vi "FYP_VI_MIDI_Test_InstrumentNote.vi"() -> ()   [LabVIEW 2013]
panel:
  in  "Pitch Note":u32=60 max=127
  in  "Velocity / Volume":u32(knob)=127 max=127 scale=0.0..127.0
  in  "stop":bool
  in  "Instrument":u32 max=127
  in  "MIDI Channel":u32 max=15
  in  "deviceID":u32
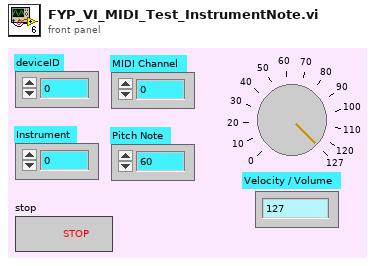
[diagram p1: front panel]
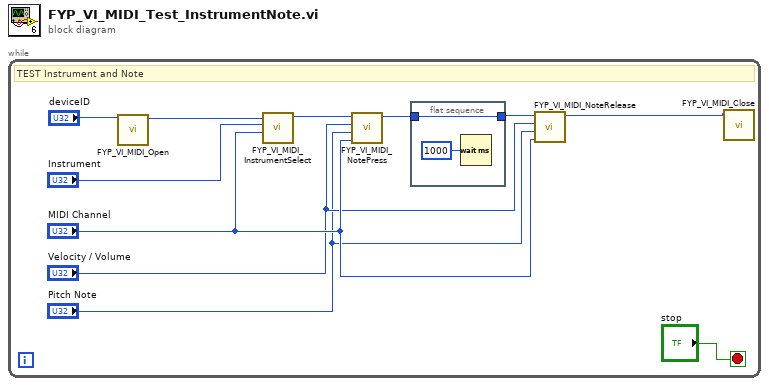
[diagram p0: block diagram]
diagram:
  n1 = while {
    stop <- "stop" stop-if-true
    # "TEST Instrument and Note"
    n2 = call "FYP_VI_MIDI_Open.vi"("deviceID"="deviceID") -> ("midiOut"=w6:i32)  [unwired: 5 in, 1 out]
    n3 = call "FYP_VI_MIDI_InstrumentSelect.vi"("MIDI Channel"="MIDI Channel", "Instrument"="Instrument", "midiOut handle"=w6) -> ("midiOut handle"=w4:i32)  [unwired: 3 in, 1 out]
    n4 = call "FYP_VI_MIDI_NotePress.vi"("MIDI Channel"="MIDI Channel", "Pitch Note"="Pitch Note", "Velocity / Volume"="Velocity / Volume", "midiOut Handle"=w4) -> ("midiOut handle"=w3:i32)  [unwired: 2 in, 1 out]
    n5 = flat-sequence {
      tunnel: w3 -> [w12]
      tunnel: [w12] -> w2
      frame #0 {
        n6 = Wait (ms)(milliseconds to wait=u32 1000) -> ()  [unwired: 1 out]
      }
    }
    n7 = call "FYP_VI_MIDI_NoteRelease.vi"("MIDI Channel"="MIDI Channel", "Pitch Note"="Pitch Note", "Velocity / Volume"="Velocity / Volume", "midiOut Handle"=w2) -> ("midiOut handle"=w5:i32)  [unwired: 2 in, 1 out]
    n8 = call "FYP_VI_MIDI_Close.vi"("midiOut"=w5) -> ()  [unwired: 6 in, 1 out]
  }
